vi "alpha Val LV.vi"(8 "error in (no error)":errorcluster, 10 "dataLength":u64, 11 "laguerreOrder":u64) -> (0 "error out":errorcluster, 3 "alpha":dbl)   [LabVIEW 2024, in "LaguerreDeconLib.lvlib"]
doc: "extern \"C\" DECONLIBRARY_API double alphaValLV(const unsigned long long laguerreOrder = 12, const unsigned long long dataLength = 680);"
uses:
  LaguerreDeconLib.lvlib
  LaguerreDeconDLL.dll
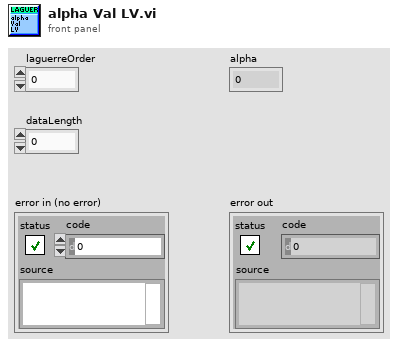
[diagram p1: front panel]
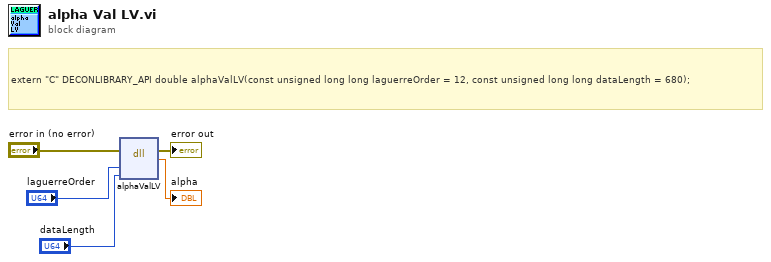
[diagram p0: block diagram]
diagram:
  # "extern \"C\" DECONLIBRARY_API double alphaValLV(const unsigned long long laguerreOrder = 12, const unsigned long long dataLength = 680);"
  n1 = dll-call lib="C:/Users/MarcuAdmin/Documents/GitHub/FLSLV/V6 APD LV/LaguerreDeconLib/LaguerreDeconDLL.*" fn="alphaValLV"(error in="error in (no error)", "laguerreOrder"="laguerreOrder", "dataLength"="dataLength") -> (error out=→"error out":errorcluster, "return type"=→"alpha":dbl)  [unwired: 4 in, 1 out]
